vi "determineClassVersion__ogtk.vi"(8 "error in (no error)":errorcluster, 10 "className":string) -> (0 "error out":errorcluster, 2 "versionNumber":u8[](array[numeric]))   [LabVIEW 2023, in "openg_variant.lvlib" / "Reflection__ogtk.lvclass"]
doc: "Given a class name, determine the version number of the input object. Version Number is formatted as a byte array.\n\nGCraftsman JSON Object Serialization Toolkit\nwww.GCraftsman.com\nCopyright (c) 2017, GCraftsman"
uses:
  Reflection__ogtk.lvclass
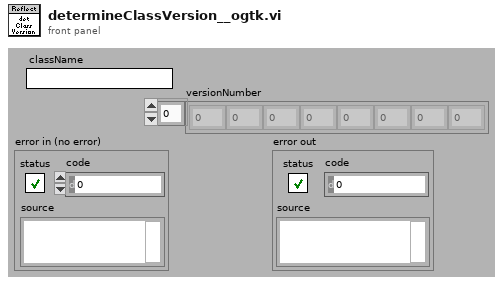
[diagram p1: front panel]
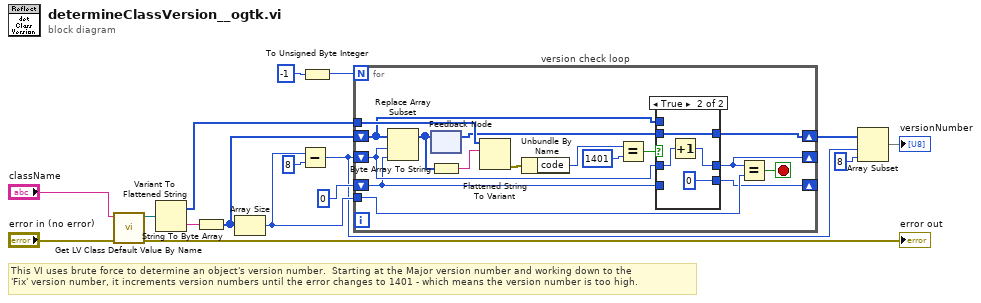
[diagram p0: block diagram]
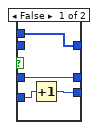
[diagram p2: hidden frame]
diagram:
  # "This VI uses brute force to determine an object's version number.  Starting at the Major version number and working down to the\n'Fix' version number, it increments version numbers until the error changes to 1401 - which means the version number is too high."
  n1 = call <vilib>:"Get LV Class Default Value By Name.vi"("error in (no error)"="error in (no error)", "class name"="className") -> ("error out"=→"error out":errorcluster, "object"=w4:refnum<class>)  [unwired: 8 in]
  n2 = Variant To Flattened String(Variant=w4) -> (data string=w15:string, 1:w13:i16[])
  n3 = String To Byte Array(string=w15) -> (unsigned byte array=w14:u8[])
  n4 = Array Size(array=w14) -> (size(s)=w10:i32)
  n5 = Subtract(x=w10, y=8) -> (x-y=w7:i32)
  n6 = To Unsigned Byte Integer(number=i8 -1) -> (unsigned 8bit integer=w11:u8)
  n7 = for "version check loop" {
    N: w11 -> [_]
    tunnel: w13 -> [w31]
    shift-right: [w23] -> w8
    shift-left: w14 -> [w27]
    shift-right: [w21] -> _
    shift-left: w7 -> [w22]
    tunnel: w10 -> [w20]
    shift-right: [w17] -> _
    shift-left: u8 0 ("unsigned 8bit integer") -> [w18]
    stop <- w19 stop-if-true
    n8 = Replace Array Subset(array=w27, new element=w18, index=w22) -> (w26:u8[])
    n9 = feedback #1() -> (w25:u8[])  [unwired: 1 in]
    n10 = feedback-in #1(w26) -> ()
    n11 = Byte Array To String(unsigned byte array=w26) -> (string=w32:string)
    n12 = Flattened String To Variant(6:w32, 7:w31) -> (0:w28:errorcluster)  [unwired: 1 in, 1 out]
    n13 = Unbundle By Name(w28) -> ("code"=w30:i32)
    n14 = Equal?(x=w30, y=1401) -> (x = y?=w24:bool)
    n15 = case shown="True" w24 {
      tunnel: w27 -> [w36 _]
      tunnel: w25 -> [_ w40]
      tunnel: [w36 w40] -> w23
      tunnel: w22 -> [w35 w39]
      tunnel: [w35 w38] -> w21
      tunnel: w18 -> [w34 _]
      tunnel: [w33 u8 0 ("unsigned 8bit integer")] -> w17
      frame False {
        n16 = Increment(x=w34) -> (x+1=w33:u8)
      }
      frame True {
        n17 = Increment(x=w39) -> (x+1=w38:i32)
      }
    }
    n18 = Equal?(x=w21, y=w20) -> (x = y?=w19:bool)
  }
  n19 = Array Subset(array=w8, index=w7, length=8) -> (→"versionNumber":u8[])
